vi "String.Selection List Change Check.vi"(9 "Sel":i32, 10 "Names":string[](array[string]), 11 "New Names":string[](array[string])) -> (0 "SelName Same":bool, 1 "Sel Out":i32, 2 "Names Out":string[](array[string]), 3 "List Change":bool)   [LabVIEW 2019]
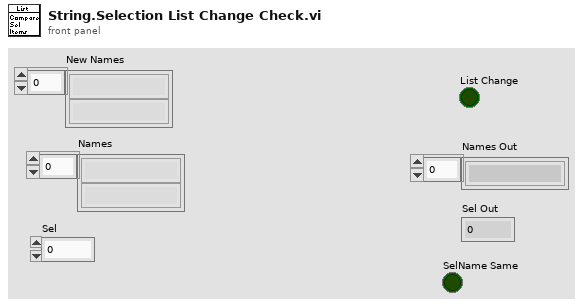
[diagram p1: front panel]
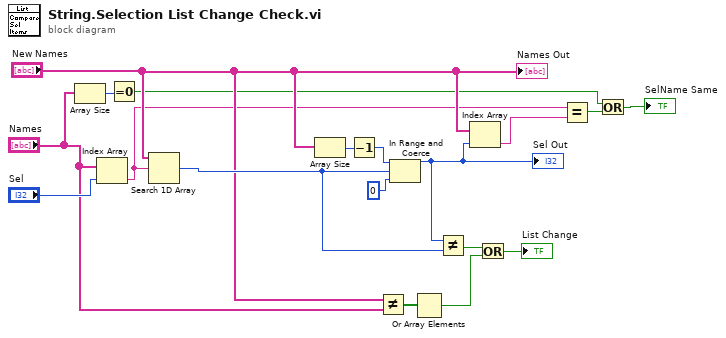
[diagram p0: block diagram]
diagram:
  n1 = Array Size(array="Names") -> (size(s)=w3:i32)
  n2 = Index Array(array="Names", index="Sel") -> (element=w7:string)
  n3 = Equal To 0?(x=w3) -> (x = 0?=w2:bool)
  n4 = Search 1D Array(1D array="New Names", element=w7) -> (index of element=w14:i32)  [unwired: 1 in]
  n5 = Array Size(array="New Names") -> (size(s)=w18:i32)
  n6 = Decrement(x=w18) -> (x-1=w17:i32)
  n7 = Not Equal?(x="New Names", y="Names") -> (x != y?=w12:bool[])
  n8 = In Range and Coerce(upper limit=w17, x=w14, lower limit=0 ("upper limit")) -> (coerced(x)=w8:i32)  [unwired: 1 out]
  "Sel Out" <- w8
  n9 = Or Array Elements(Boolean array=w12) -> (logical OR=w11:bool)
  n10 = Not Equal?(x=w8, y=w14) -> (x != y?=w13:bool)
  n11 = Index Array(array="New Names", index=w8) -> (element=w6:string)
  n12 = Or(x=w13, y=w11) -> (x .or. y?=→"List Change":bool)
  n13 = Equal?(x=w7, y=w6) -> (x = y?=w5:bool)
  n14 = Or(x=w2, y=w5) -> (x .or. y?=→"SelName Same":bool)
  "Names Out" <- "New Names"
